vi "Allow Window Resize.vi"(8 "error in (no error)":errorcluster, 10 "Allow Resize?":bool, 11 "Hwnd":u32) -> (0 "error out":errorcluster)   [LabVIEW 2011]
doc: "This VI will allow or not allow a window to be resized. The windows <b>Hwnd</b> is needed.\n\nAfter allowing or not allowing the resize, the window may need to have the redraw method to appear properly."
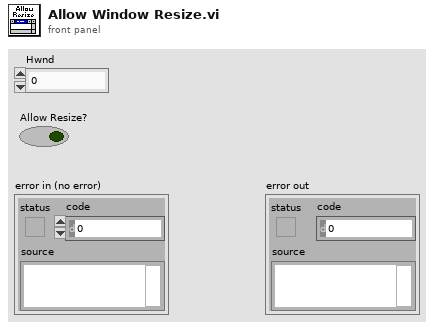
[diagram p1: front panel]
types:
  T1 = enum16{"WS_BORDER", "WS_CAPTION", "WS_CHILD", "WS_CLIPCHILDREN", "WS_CLIPSIBLINGS", "WS_DISABLED", "WS_DLGFRAME", "WS_HSCROLL", "WS_MAXIMIZE", "WS_MAXIMIZEBOX", "WS_MINIMIZE", "WS_MINIMIZEBOX", "WS_OVERLAPPED", "WS_POPUP", "WS_SYSMENU", "WS_THICKFRAME", "WS_VISIBLE", "WS_VSCROLL"}
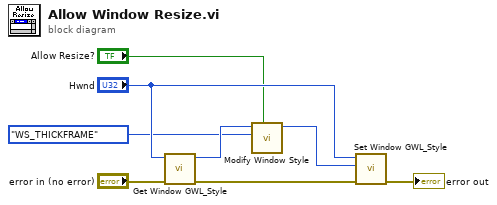
[diagram p0: block diagram]
diagram:
  n1 = call "Get Window GWL_Style.vi"("error in (no error)"="error in (no error)", "Hwnd"="Hwnd") -> ("error out"=w8:errorcluster, "Style"=w4:u32)  [unwired: 8 in]
  n2 = call "Modify Window Style.vi"("Style Value"="Allow Resize?", "GWL_Style Modify"=T1."WS_THICKFRAME", "GWL_Style In"=w4) -> ("GWL_Style Out"=w1:u32)  [unwired: 7 in, 1 out]
  n3 = call "Set Window GWL_Style.vi"("error in (no error)"=w8, "Style"=w1, "Hwnd"="Hwnd") -> ("error out"=→"error out":errorcluster)  [unwired: 8 in]
